vi "GlobalPlotData7.vi"(0 "Function select":string, 1 "# Plot points":u32, 2 "IO data point in":cluster{"Time":u32, "Value":sgl}, 3 "Data channel #":u32, 4 "# Data channels":u32) -> (5 "Single data plot cluster":cluster{"Array":u32[], "Array 2":sgl[]})   [LabVIEW 2013]
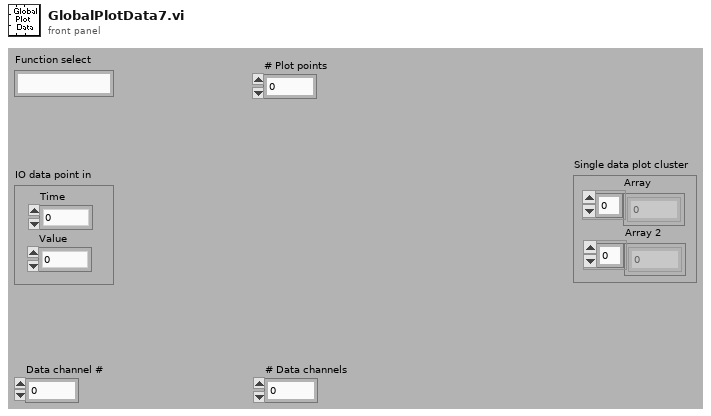
[diagram p1: front panel]
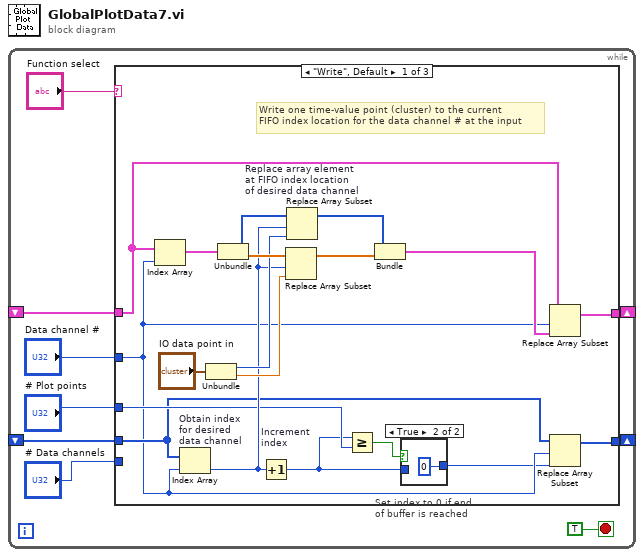
[diagram p0: block diagram]
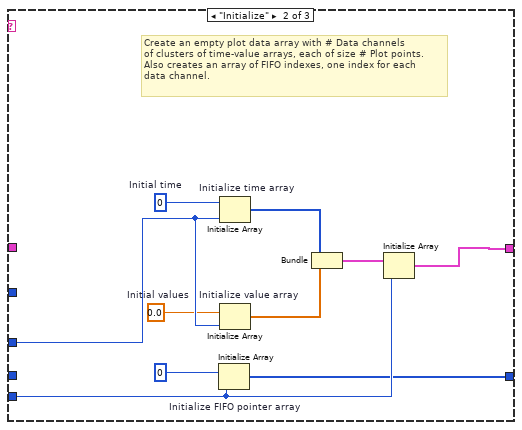
[diagram p3: hidden frame]
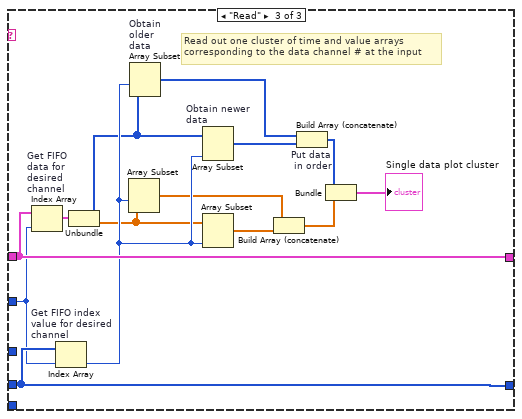
[diagram p4: hidden frame]
diagram:
  n1 = while {
    shift-right: [w7] -> _
    shift-left: _ -> [w6]
    shift-right: [w2] -> _
    shift-left: _ -> [w1]
    stop <- TRUE stop-if-true
    n2 = case shown="\"Write\", Default" "Function select" {
      tunnel: "# Plot points" -> [w20 w40 _]
      tunnel: [w28 w32 w54] -> w7
      tunnel: w6 -> [w13 _ w54]
      tunnel: "Data channel #" -> [w11 _ w52]
      tunnel: "# Data channels" -> [_ w33 _]
      tunnel: [w12 w31 w53] -> w2
      tunnel: w1 -> [w17 _ w53]
      frame "Write", Default {
        # "Write one time-value point (cluster) to the current\nFIFO index location for the data channel # at the input"
        n3 = Index Array(array=w13, index=w11) -> (element=w27:cluster{u32[], sgl[]})
        n4 = Index Array "Obtain index\nfor desired\ndata channel"(array=w17, index=w11) -> (element=w21:i32)
        n5 = Unbundle("IO data point in") -> ("Time"=w23:u32, "Value"=w22:sgl)
        n6 = Unbundle(w27) -> (w25:u32[], w24:sgl[])
        n7 = Increment "Increment\nindex"(x=w21) -> (x+1=w18:i32)
        n8 = Replace Array Subset(array=w24, new element=w22, index=w21) -> (w15:sgl[])
        n9 = Replace Array Subset "Replace array element\nat FIFO index location\nof desired data channel"(array=w25, new element=w23, index=w21) -> (w16:u32[])
        n10 = Greater Or Equal?(x=w18, y=w20) -> (x >= y?=w19:bool)
        n11 = Bundle(w16, w15) -> (w14:cluster{u32[], sgl[]})  [unwired: 1 in]
        n12 = case "Set index to 0 if end\nof buffer is reached" shown="True" w19 {
          tunnel: [w29 0] -> w10
          tunnel: w18 -> [w29 _]
          frame False {
          }
          frame True {
          }
        }
        n13 = Replace Array Subset(array=w13, new element=w14, index=w11) -> (w28:cluster{u32[], sgl[]}[])
        n14 = Replace Array Subset(array=w17, new element=w10, index=w11) -> (w12:i32[])
      }
      frame "Initialize" {
        w38 = u32 0  # Initial time
        w39 = sgl 0.0  # Initial values
        # "Create an empty plot data array with # Data channels\nof clusters of time-value arrays, each of size # Plot points.\nAlso creates an array of FIFO indexes, one index for each\ndata channel."
        n15 = Initialize Array "Initialize FIFO pointer array"(0, w33) -> (w31:i32[])
        n16 = Initialize Array "Initialize time array"(w38, w40) -> (w35:u32[])
        n17 = Initialize Array "Initialize value array"(w39, w40) -> (w36:sgl[])
        n18 = Bundle(w35, w36) -> (w34:cluster{u32[], sgl[]})  [unwired: 1 in]
        n19 = Initialize Array(w34, w33) -> (w32:cluster{u32[], sgl[]}[])
      }
      frame "Read" {
        # "Read out one cluster of time and value arrays\ncorresponding to the data channel # at the input"
        n20 = Index Array "Get FIFO\ndata for\ndesired\nchannel"(array=w54, index=w52) -> (element=w51:cluster{u32[], sgl[]})
        n21 = Index Array "Get FIFO index\nvalue for desired\nchannel"(array=w53, index=w52) -> (element=w50:i32)
        n22 = Unbundle(w51) -> (w47:u32[], w42:sgl[])
        n23 = Array Subset(array=w42, index=w50) -> (w44:sgl[])  [unwired: 1 in]
        n24 = Array Subset "Obtain\nolder\ndata"(array=w47, index=w50) -> (w49:u32[])  [unwired: 1 in]
        n25 = Array Subset "Obtain newer \ndata"(array=w47, length=w50) -> (w48:u32[])  [unwired: 1 in]
        n26 = Array Subset(array=w42, length=w50) -> (w43:sgl[])  [unwired: 1 in]
        n27 = Build Array (concatenate)(w44, w43) -> (w41:sgl[])
        n28 = Build Array (concatenate) "Put data\n in order"(w49, w48) -> (w46:u32[])
        n29 = Bundle(w46, w41) -> (→"Single data plot cluster":cluster{u32[], sgl[]})  [unwired: 1 in]
      }
    }
  }
